vi "demo - Simple Serial with conversion.vi"() -> ()   [LabVIEW 2024]
doc: "#vi_description \nSends a simple serial request and receives a response as as string of byte characters.\nModified NI Example.\nThetic Engineering Ltd."
uses:
  <vilib>/Instr/_visa.llb/VISA Configure Serial Port (Instr).vi
  Serial - Settings.ctl
panel:
  out "output cluster":T1
  out "timestamp":timestamp
  out "firmware":string
  out "array data":string[](array[string])
  in  "Serial Settings":T2={"baud rate"=9600, "data bits"=8, "parity"=enum."None", "stop bits"=10, "flow control"=0} {"flow control" items=["None"=0, "XON/XOFF"=1, "RTS/CTS"=2, "DTR/DSR"=4]; "stop bits" items=["1.0"=10, "1.5"=15, "2.0"=20]; "data bits" min=5 max=8 step=1; "baud rate" items=["75"=75, "110"=110, "134"=134, "150"=150, "300"=300, "600"=600, "1200"=1200, "1800"=1800, "2400"=2400, "4800"=4800, "7200"=7200, "9600"=9600, "14400"=14400, "19200"=19200, "28800"=28800, "38400"=38400, "56000"=56000, "57600"=57600, "115200"=115200, "128000"=128000, "230400"=230400]}
  out "bytes read":u32
  in  "delay before read (ms)":u32=500
  out "Response":string
  in  "VISA resource name":refnum<visa-resource-name>="COM3"
  # "Multi-stage method"
  # "Single stage method"
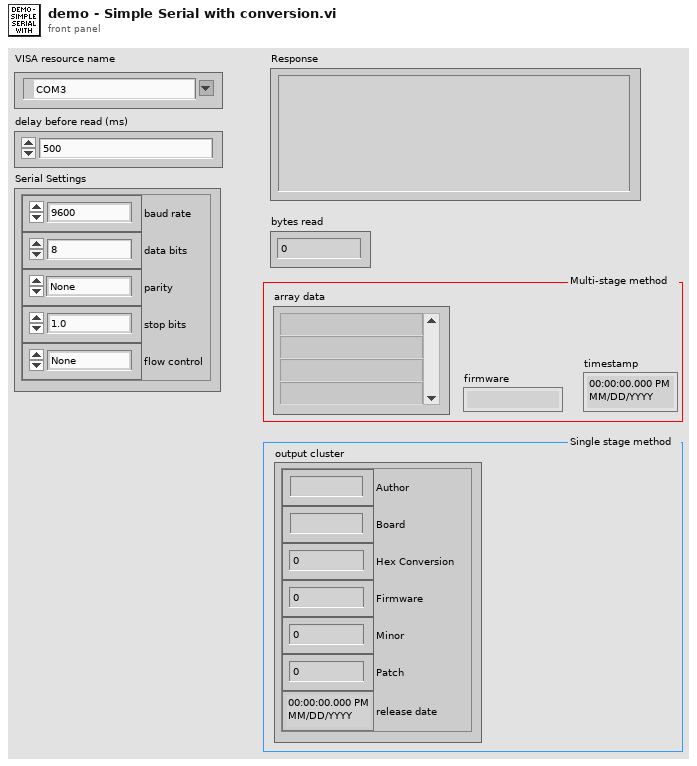
[diagram p1: front panel]
types:
  T1 = cluster{"Author":string, "Board":string, "Hex Conversion":u32, "Firmware":i32, "Minor":i32, "Patch":i32, "release date":timestamp}
  T2 = typedef "Serial - Settings.ctl" = cluster{"baud rate":u32, "data bits":u16, "parity":enum16{"None", "Odd", "Even", "Mark", "Space"}, "stop bits":u16, "flow control":u16}
  T3 = cluster{string, string, u32, i32, i32, i32, timestamp}
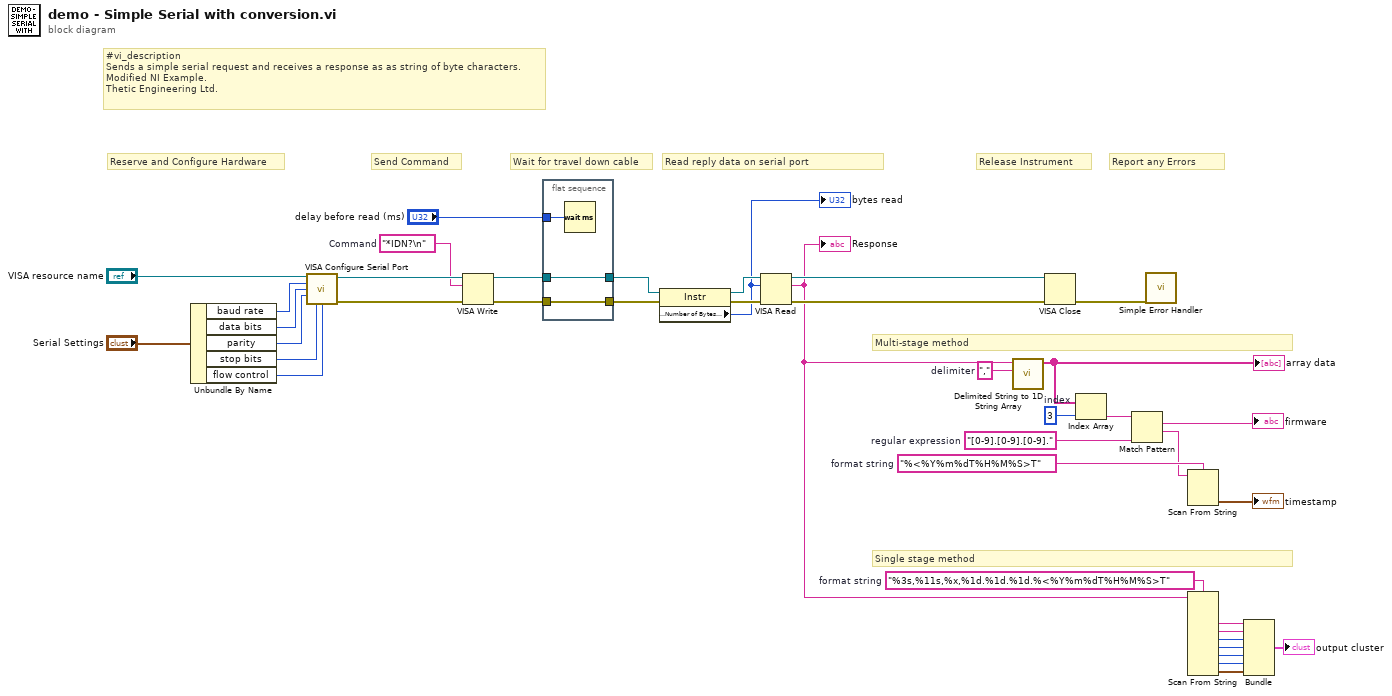
[diagram p0: block diagram]
diagram:
  w10 = "%3s,%11s,%x,%1d.%1d.%1d.%<%Y%m%dT%H%M%S>T"  # format string
  w13 = "%<%Y%m%dT%H%M%S>T"  # format string
  w16 = "[0-9].[0-9].[0-9]."  # regular expression
  w18 = 3  # index
  w14 = ","  # delimiter
  w29 = "*IDN?\n"  # Command
  # "Single stage method"
  # "Multi-stage method"
  # "Report any Errors"
  # "Release Instrument"
  # "Read reply data on serial port"
  # "Wait for travel down cable"
  # "Send Command"
  # "Reserve and Configure Hardware"
  # "#vi_description \nSends a simple serial request and receives a response as as string of byte characters.\nModified NI Example.\nThetic Engineering Ltd."
  n1 = Unbundle By Name("Serial Settings") -> ("baud rate"=w24:u32, "data bits"=w23:u16, "parity"=w22:enum16{"None", "Odd", "Even", "Mark", "Space"}, "stop bits"=w21:u16, "flow control"=w20:u16)
  n2 = call-poly "VISA Configure Serial Port"("VISA resource name"="VISA resource name", "baud rate (9600)"=w24, "data bits (8)"=w23, "parity (0:none)"=w22, "stop bits (10: 1 bit)"=w21, "flow control (0:none)"=w20) -> ("VISA resource name out"=w38:refnum<visa-resource-name>, "error out"=w39:errorcluster)  [unwired: 3 in, 5 out]
  n3 = VISA Write(VISA resource name=w38, write buffer=w29, error in (no error)=w39) -> (VISA resource name out=w32:refnum<visa-resource-name>, error out=w34:errorcluster)  [unwired: 1 out]
  n4 = flat-sequence {
    tunnel: w34 -> [w42]
    tunnel: [w42] -> w33
    tunnel: w32 -> [w41]
    tunnel: [w41] -> w31
    tunnel: "delay before read (ms)" -> [w43]
    frame #0 {
      n5 = Wait (ms)(milliseconds to wait=w43) -> ()  [unwired: 1 out]
    }
  }
  n6 = property on="Property Node" class="Instr"(reference=w31, error in=w33) -> (reference out=w28:refnum<visa-resource-name>, error out=w27:errorcluster, "Serial Settings:Number of Bytes at Serial Port"=w26:u32)
  "bytes read" <- w26
  n7 = VISA Read(VISA resource name=w28, byte count=w26, error in (no error)=w27) -> (VISA resource name out=w36:refnum<visa-resource-name>, read buffer=w2:string, error out=w37:errorcluster)  [unwired: 1 out]
  "Response" <- w2
  n8 = call <vilib>:"Delimited String to 1D String Array.vi"("delimiter"=w14, "delimited string"=w2) -> ("string array"=w19:string[])  [unwired: 9 in]
  "array data" <- w19
  n9 = VISA Close(VISA resource name=w36, error in (no error)=w37) -> (error out=w35:errorcluster)
  n10 = Index Array "Index Array"(array=w19, index=w18) -> (element=w17:string)
  n11 = Match Pattern(string=w17, regular expression=w16) -> (match substring=→"firmware":string, after substring=w12:string)  [unwired: 1 in, 2 out]
  n12 = call <vilib>:"Simple Error Handler.vi"("error in (no error)"=w35) -> ()  [unwired: 1 in, 8 out]
  n13 = Scan From String "Scan From String"(format string=w13, input string=w12) -> (output 1=→"timestamp":timestamp)  [unwired: 3 in, 3 out]
  n14 = Scan From String "Scan From String"(format string=w10, input string=w2) -> (output 1=w9:string, output 2=w8:string, output 3=w7:u32, output 4=w6:i32, output 5=w5:i32, output 6=w4:i32, output 7=w3:timestamp)  [unwired: 9 in, 3 out]
  n15 = Bundle(w9, w8, w7, w6, w5, w4, w3) -> (→"output cluster":T3)  [unwired: 1 in]
